vi "applyInsertSpaceY.vi"(4 "deltaY":u16, 8 "error in (no error)":errorcluster, 10 "originY":i32, 11 "Wire in":refnum<class "Wire.lvclass">) -> (0 "error out":errorcluster, 3 "Wire out":refnum<class "Wire.lvclass">)   [LabVIEW 2023, in "TLC_Scripto.lvlib" / "Wire.lvclass"]
uses:
  Wire.lvclass
  Wire.lvclass/Wire.ctl
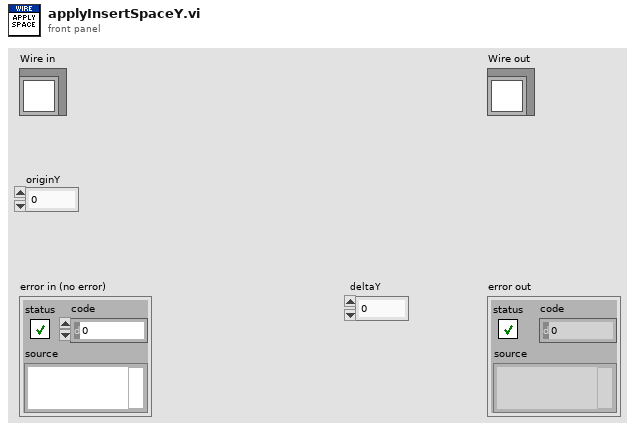
[diagram p1: front panel]
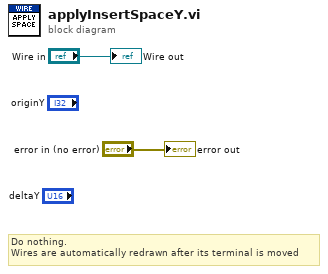
[diagram p0: block diagram]
diagram:
  # "Do nothing.\nWires are automatically redrawn after its terminal is moved"
  "error out" <- "error in (no error)"
  "Wire out" <- "Wire in"
